vi "Calibration.vi"() -> ()   [LabVIEW 2009]
uses:
  lib/Apps/On Off Button.ctl
  CalibrationRampState.ctl
  Calibration Readings.ctl
  DAQ Read Actions.ctl
  <vilib>/DAQmx/write.llb/DAQmx Write (Analog 1D DBL NChan 1Samp).vi
panel:
  in  "Readings":T1
  in  "Actuator":i32(listbox)
  out "Readings":T2(graph)
  out "Ramp State":T3
  in  "Execute":bool
  in  "Logging":T4
  out "Command Voltage":dbl[](array[numeric])
  in  "Log File Path":path=path "C:/Documents and Settings/mbletzin/Desktop/CalVolts.txt"
  in  "Ramp Voltage":dbl[](array[numeric])
  out "Control Voltage":dbl[](array[numeric])
  in  "rate":dbl=50.0
  in  "samples per channel":i32=30
  out "Servo Error Reading":dbl[](array[numeric])
  in  "Command Voltage Task":refnum<k21>="Command Voltages"
  in  "Readings Task":refnum<k21>="All Readings"
  in  "Write error in (no error)":errorcluster
  out "Read error out":errorcluster
  out "Write error out":errorcluster
  in  "Read error in (no error)":errorcluster
  out "Load Cell \nReading":dbl[](array[numeric])
  out "LVDT Reading":dbl[](array[numeric])
  in  "Command Voltage Input":T5={"Actuator X1"=0.0, "Actuator Z1"=0.0, "Actuator Y1"=0.0, "Actuator X2"=0.0, "Actuator Z3"=0.0, "Actuator Z2"=0.0, "Ramp Time"=30.0, "No. of Steps"=100} {"Actuator Z2" min=-10.0 max=10.0 step=0.1 scale=-10.0..10.0; "Actuator Z3" min=-10.0 max=10.0 step=0.1 scale=-10.0..10.0; "Actuator X2" min=-10.0 max=10.0 step=0.1 scale=-10.0..10.0; "Actuator Y1" min=-10.0 max=10.0 step=0.1 scale=-10.0..10.0; "Actuator Z1" min=-10.0 max=10.0 step=0.1 scale=-10.0..10.0; "Actuator X1" min=-10.0 max=10.0 step=0.1 scale=-10.0..10.0}
  in  "Quit":bool
  # "LBCB CALIBRATION PROGRAM"
  # "Channel Order:\nX1 X2 Y1 Z1 Z2 Z3\n\nLVDT Readings\nLoadcell Readings\nServo Errors"
  # "Channel Order:\nX1 X2 Y1 Z1 Z2 Z3"
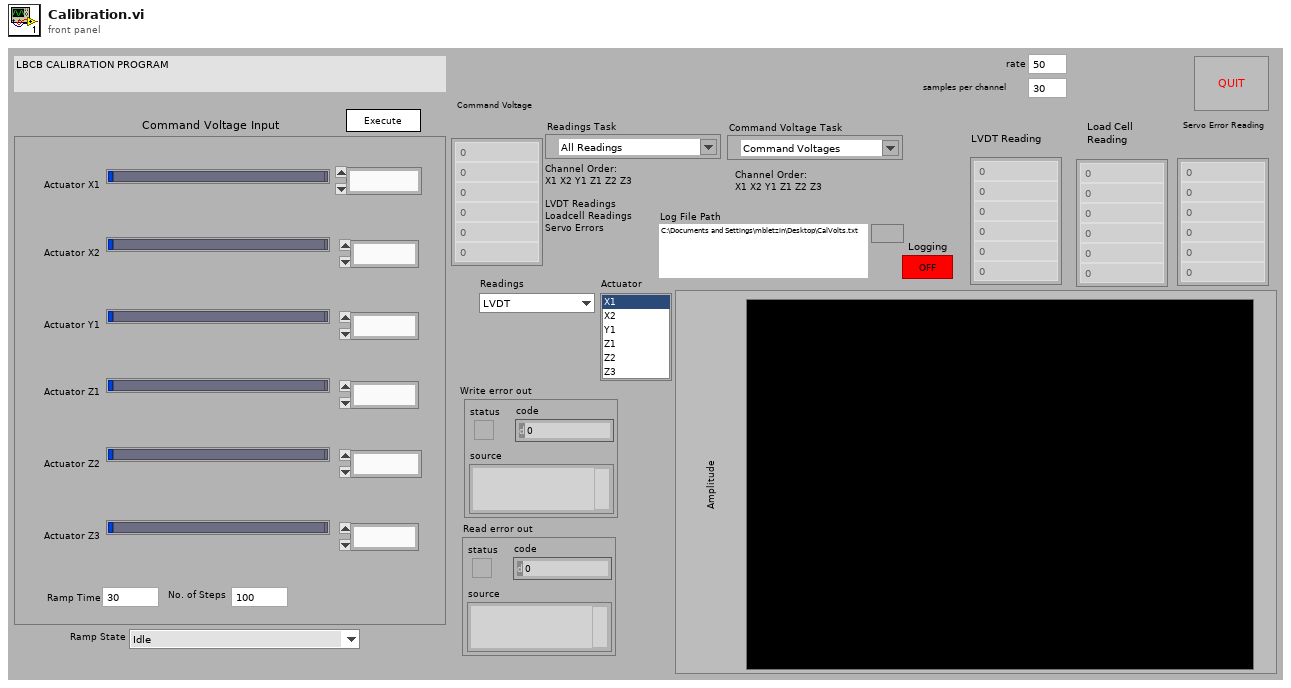
[diagram p1: front panel]
types:
  T1 = typedef "Calibration Readings.ctl" = enum16{"LVDT", "Load Cell", "Servo Errors"}
  T2 = cluster{"Average[0]":dbl, "Average[1]":dbl, "Average[2]":dbl, "Average[3]":dbl, "Average[4]":dbl, "Average[5]":dbl, "Average[6]":dbl, "Average[7]":dbl, "Average[8]":dbl}
  T3 = typedef "CalibrationRampState.ctl" = enum16{"Idle", "Start Ramp", "Ramping"}
  T4 = typedef "On Off Button.ctl" = bool
  T5 = cluster{"Actuator X1":dbl, "Actuator Z1":dbl, "Actuator Y1":dbl, "Actuator X2":dbl, "Actuator Z3":dbl, "Actuator Z2":dbl, "Ramp Time":dbl, "No. of Steps":i32}
  T6 = typedef "DAQ Read Actions.ctl" = enum16{"Start", "Read", "Stop"}
  T7 = cluster{"Average[0]":dbl, "Average[1]":dbl, "Average[2]":dbl, "Average[3]":dbl, "Average[4]":dbl, "Average[5]":dbl, "Average[6]":dbl, "Average[7]":dbl, "Average[8]":dbl}[]
  T8 = enum16{"open", "replace", "create", "open or create", "replace or create", "replace or create with confirmation"}
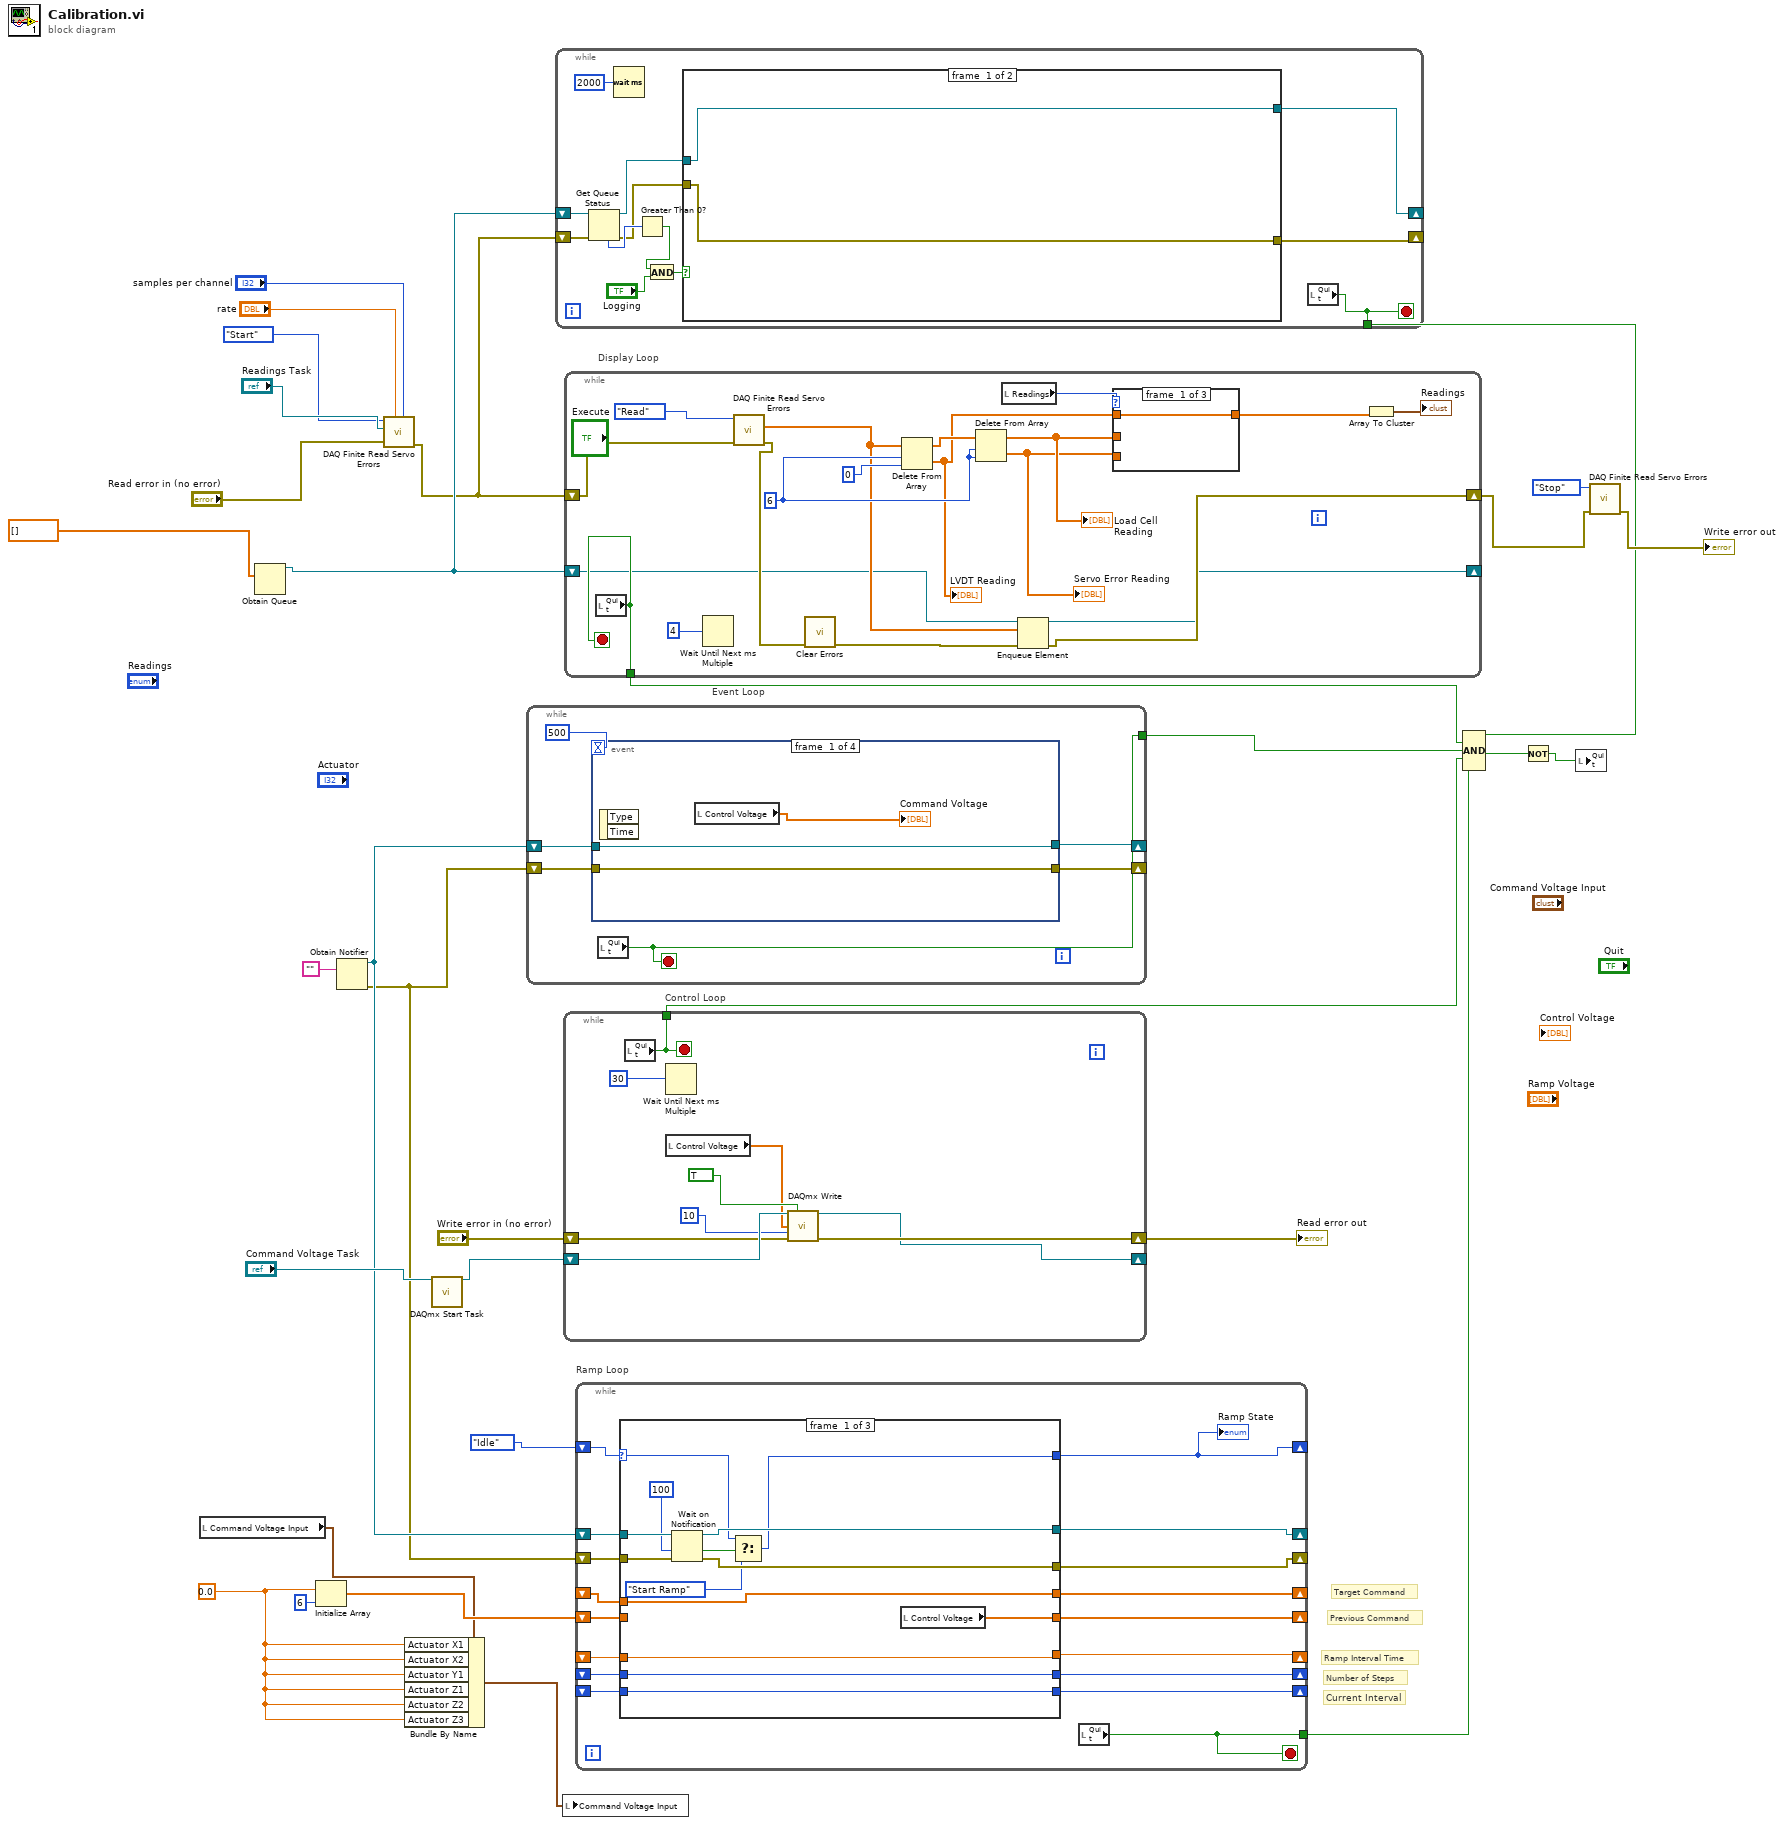
[diagram p0: block diagram]
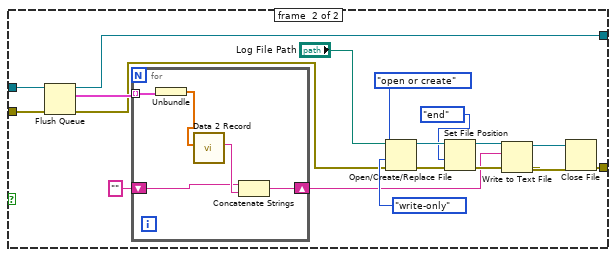
[diagram p2: hidden frame]
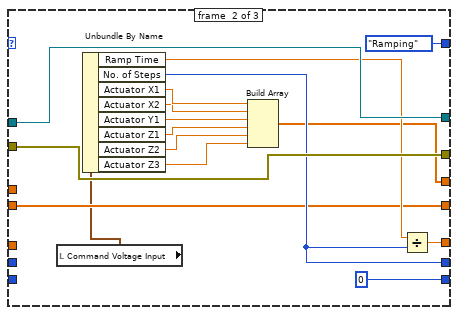
[diagram p3: hidden frame]
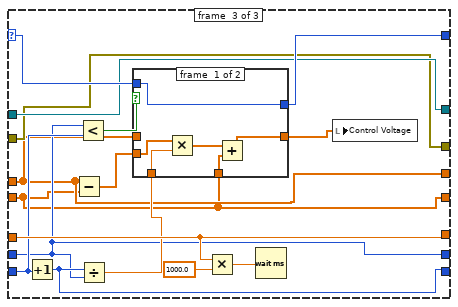
[diagram p4: hidden frame]
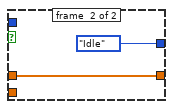
[diagram p5: hidden frame]
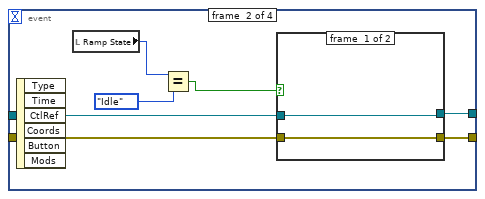
[diagram p6: hidden frame]
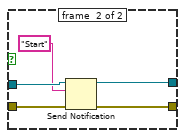
[diagram p7: hidden frame]
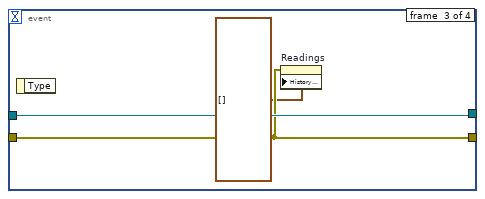
[diagram p8: hidden frame]
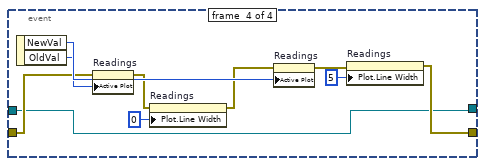
[diagram p9: hidden frame]
diagram:
  w1 = 0.0 ("element")
  # "Previous Command"
  # "Target Command"
  # "Ramp Interval Time"
  # "Number of Steps"
  # "Current Interval"
  n1 = local read "Command Voltage Input"() -> (w2:T5)
  n2 = Obtain Queue(element data type=dbl[] []) -> (queue out=w8:refnum<queue>)  [unwired: 4 in, 2 out]
  n3 = Initialize Array(w1, 6 ("dimension size")) -> (w4:dbl[])
  n4 = Obtain Notifier(notification data type="") -> (notifier out=w12:refnum<notifier>, error out=w11:errorcluster)  [unwired: 3 in, 1 out]
  n5 = call "DAQ Finite Read Servo Errors.vi"("samples per channel"="samples per channel", "rate"="rate", "error in"="Read error in (no error)", "task/channels in"="Readings Task", "Action"=DAQ_Read_Actions."Start") -> ("error out"=w7:errorcluster)  [unwired: 6 out]
  n6 = Bundle By Name(cluster=w2, "Actuator X1"=w1, "Actuator X2"=w1, "Actuator Y1"=w1, "Actuator Z1"=w1, "Actuator Z2"=w1, "Actuator Z3"=w1) -> (w3:T5)
  n7 = call <vilib>:"DAQmx Start Task.vi"("task/channels in"="Command Voltage Task") -> ("task out"=w31:refnum<k21>)  [unwired: 1 in, 13 out]
  n8 = while "Event Loop" {
    tunnel: [w36] -> w27
    shift-right: [w32] -> _
    shift-left: w11 -> [w34]
    shift-right: [w33] -> _
    shift-left: w12 -> [w35]
    stop <- w36 stop-if-true
    n9 = event shown="[2] \"Readings\": Value Change" {
      selector: _ -> [_ _ _ _]
      dyn-events: _ -> [_ _ _ _]
      timeout: 500 -> [_ _ _ _]
      tunnel: w35 -> [w40 w45 w57 w59]
      tunnel: w34 -> [w39 w44 w56 w64]
      tunnel: [w40 w43 w57 w59] -> w33
      tunnel: [w39 w42 w56 w60] -> w32
      event #0 {
        n10 = event-data() -> ()  [unwired: 3 out]
        n11 = local read "Control Voltage"() -> (→"Command Voltage":dbl[])
      }
      event #1 {
        n12 = event-data() -> ()  [unwired: 7 out]
        n13 = local read "Ramp State"() -> (w41:T3)
        n14 = Equal?(x=w41, y=enum16{"Idle", "Start Ramp", "Ramping"}."Idle") -> (x = y?=w46:bool)
        n15 = case shown="True" w46 {
          tunnel: w45 -> [w49 w54]
          tunnel: w44 -> [w48 w52]
          tunnel: [w49 w51] -> w43
          tunnel: [w48 w50] -> w42
          frame #0 {
          }
          frame #1 {
            n16 = Send Notification(notification="Start", notifier=w54, error in (no error)=w52) -> (notifier out=w51:refnum<notifier>, error out=w50:errorcluster)
          }
        }
      }
      event #2 {
        n17 = event-data() -> ()  [unwired: 2 out]
        n18 = property on="Readings" class="WFChart (strict)"(error in=w56, "History Data"=T7 []) -> ()  [unwired: 1 in, 2 out]
      }
      event #3 {
        n19 = event-data() -> ("NewVal"=w67:i32, "OldVal"=w66:i32)  [unwired: 1 out]
        n20 = property on="Readings" class="WFChart (strict)"(error in=w64, "Active Plot"=w66) -> (error out=w65:errorcluster)  [unwired: 1 in, 1 out]
        n21 = property on="Readings" class="WFChart (strict)"(error in=w65, "Plot.Line Width"=u8 0) -> (error out=w62:errorcluster)  [unwired: 1 in, 1 out]
        n22 = property on="Readings" class="WFChart (strict)"(error in=w62, "Active Plot"=w67) -> (error out=w61:errorcluster)  [unwired: 1 in, 1 out]
        n23 = property on="Readings" class="WFChart (strict)"(error in=w61, "Plot.Line Width"=u8 5) -> (error out=w60:errorcluster)  [unwired: 1 in, 1 out]
      }
    }
    n24 = local read "Quit"() -> (w36:bool)
  }
  n25 = while {
    shift-right: [w73] -> _
    shift-left: w8 -> [w79]
    shift-right: [w74] -> _
    shift-left: w7 -> [w78]
    tunnel: [w72] -> w6
    stop <- w72 stop-if-true
    n26 = Get Queue Status(queue=w79, error in (no error)=w78) -> (queue out=w76:refnum<queue>, error out=w75:errorcluster, # elements in queue=w77:i32)  [unwired: 1 in, 5 out]
    n27 = Wait (ms)(milliseconds to wait=u32 2000) -> ()  [unwired: 1 out]
    n28 = Greater Than 0?(x=w77) -> (x > 0?=w69:bool)
    n29 = And(x=w69, y="Logging") -> (x .and. y?=w70:T4)
    n30 = case shown="False" w70 {
      tunnel: w76 -> [w81 w89]
      tunnel: w75 -> [w80 w88]
      tunnel: [w80 w87] -> w74
      tunnel: [w81 w85] -> w73
      frame #0 {
      }
      frame #1 {
        n31 = Flush Queue(queue=w89, error in (no error)=w88) -> (queue out=w85:refnum<queue>, remaining elements=w86:cluster{dbl[]}[], error out=w84:errorcluster)
        n32 = for {
          tunnel: w86 -> [w104] mode=indexing
          shift-right: [w101] -> w83
          shift-left: "" -> [w100]
          n33 = Unbundle(w104) -> (w103:dbl[])
          n34 = call "Data 2 Record.vi"("Data"=w103) -> ("Records"=w102:string)  [unwired: 10 in]
          n35 = Concatenate Strings(w100, w102) -> (w101:string)
        }
        n36 = Open/Create/Replace File(file path (use dialog)="Log File Path", error in=w84, operation (0:open)=T8."open or create", access (0:read/write)=enum16{"read/write", "read-only", "write-only"}."write-only") -> (refnum out=w95:refnum<file>, error out=w94:errorcluster)  [unwired: 3 out]
        n37 = Set File Position(refnum=w95, from (0:start)=enum16{"start", "end", "current"}."end", error in=w94) -> (refnum out=w92:refnum<file>, error out=w93:errorcluster)  [unwired: 1 out]
        n38 = Write to Text File(file (use dialog)=w92, text=w83, error in=w93) -> (refnum out=w97:refnum<file>, error out=w98:errorcluster)  [unwired: 2 out]
        n39 = Close File(refnum=w97, error in=w98) -> (error out=w87:errorcluster)  [unwired: 1 out]
      }
    }
    n40 = local read "Quit"() -> (w72:bool)
  }
  n41 = local write "Command Voltage Input"(w3) -> ()
  n42 = while "Control Loop" {
    shift-right: [w110] -> _
    shift-left: w31 -> [w113]
    shift-right: [w111] -> w29
    shift-left: "Write error in (no error)" -> [w112]
    tunnel: [w106] -> w23
    stop <- w106 stop-if-true
    n43 = local read "Quit"() -> (w106:bool)
    n44 = Wait Until Next ms Multiple(millisecond multiple=30) -> ()  [unwired: 1 out]
    n45 = local read "Control Voltage"() -> (w105:dbl[])
    n46 = call-poly <vilib>:"DAQmx Write.vi"("task/channels in"=w113, "auto start"=TRUE, "data"=w105, "timeout"=10, "error in"=w112) -> ("task out"=w110:refnum<k21>, "error out"=w111:errorcluster)  [unwired: 9 out]
  }
  "Read error out" <- w29
  n47 = while "Display Loop" {
    shift-right: [w123] -> w17
    shift-left: w7 -> [w127]
    tunnel: [w131] -> w25
    shift-right: [w120] -> _
    shift-left: w8 -> [w121]
    stop <- w131 stop-if-true
    w129 = 6
    n48 = local read "Quit"() -> (w131:bool)
    n49 = Wait Until Next ms Multiple(millisecond multiple=4) -> ()  [unwired: 1 out]
    n50 = call "DAQ Finite Read Servo Errors.vi"("error in"=w127, "Action"=DAQ_Read_Actions."Read") -> ("error out"=w126:errorcluster, "Average"=w122:dbl[])  [unwired: 3 in, 5 out]
    n51 = call <vilib>:"Clear Errors.vi"("error in (no error)"=w126) -> ("error out"=w124:errorcluster)  [unwired: 6 out]
    n52 = Delete From Array(array=w122, length=w129, index=0) -> (deleted portion=w118:dbl[], array with subset deleted=w130:dbl[])
    "LVDT Reading" <- w118
    n53 = Delete From Array(array=w130, length=w129, index=w129) -> (deleted portion=w116:dbl[], array with subset deleted=w117:dbl[])
    "Load Cell \nReading" <- w117
    "Servo Error Reading" <- w116
    n54 = local read "Readings"() -> (w119:T1)
    n55 = Enqueue Element(queue=w121, element=w122, error in (no error)=w124) -> (queue out=w120:refnum<queue>, error out=w123:errorcluster)  [unwired: 1 in, 1 out]
    n56 = case shown="\"Servo Errors\"" w119 {
      tunnel: w118 -> [w133 _ _]
      tunnel: w117 -> [_ w134 _]
      tunnel: w116 -> [_ _ w135]
      tunnel: [w133 w134 w135] -> w115
      frame #0 {
      }
      frame #1 {
      }
      frame #2 {
      }
    }
    n57 = Array To Cluster(array=w115) -> (cluster=→"Readings":T2)
  }
  n58 = while "Ramp Loop" {
    shift-right: [w136] -> _
    shift-left: CalibrationRampState."Idle" ("Ramp State") -> [w152]
    shift-right: [w149] -> _
    shift-left: w12 -> [w151]
    shift-right: [w148] -> _
    shift-left: w11 -> [w150]
    shift-right: [w147] -> _
    shift-left: _ -> [w139]
    shift-right: [w145] -> _
    shift-left: _ -> [w140]
    shift-right: [w146] -> _
    shift-left: _ -> [w141]
    shift-right: [w144] -> _
    shift-left: w4 -> [w142]
    shift-right: [w143] -> _
    shift-left: _ -> [w138]
    tunnel: [w137] -> w10
    stop <- w137 stop-if-true
    n59 = case shown="\"Start Ramp\"" w152 {
      selector: w152 -> [w160 _ w188]
      tunnel: w151 -> [w166 w181 w186]
      tunnel: w150 -> [w165 w182 w185]
      tunnel: [w162 w181 w186] -> w149
      tunnel: [w161 w182 w185] -> w148
      tunnel: [w159 CalibrationRampState."Ramping" ("f") w187] -> w136
      tunnel: [w155 w178 w196] -> w147
      tunnel: [w153 0 w195] -> w146
      tunnel: [w154 w176 w189] -> w145
      tunnel: [w157 w168 w183] -> w144
      tunnel: [w156 w169 w184] -> w143
      tunnel: w142 -> [_ w168 w183]
      tunnel: w141 -> [w153 _ w190]
      tunnel: w140 -> [w154 _ w189]
      tunnel: w139 -> [w155 _ w196]
      tunnel: w138 -> [w156 _ w184]
      frame #0 {
        n60 = Wait on Notification(notifier=w166, timeout in ms (-1)=100, error in (no error)=w165) -> (notifier out=w162:refnum<notifier>, timed out?=w163:bool, error out=w161:errorcluster)  [unwired: 1 in, 1 out]
        n61 = Select(t=w160, s=w163, f=CalibrationRampState."Start Ramp") -> (s? t:f=w159:T3)
        n62 = local read "Control Voltage"() -> (w157:dbl[])
      }
      frame #1 {
        n63 = local read "Command Voltage Input"() -> (w167:T5)
        n64 = Unbundle By Name(w167) -> ("Ramp Time"=w179:dbl, "No. of Steps"=w176:i32, "Actuator X1"=w175:dbl, "Actuator X2"=w174:dbl, "Actuator Y1"=w173:dbl, "Actuator Z1"=w172:dbl, "Actuator Z2"=w171:dbl, "Actuator Z3"=w170:dbl)
        n65 = Build Array(w175, w174, w173, w172, w171, w170) -> (w169:dbl[])
        n66 = Divide(x=w179, y=w176) -> (x/y=w178:dbl)
      }
      frame #2 {
        n67 = Increment(x=w190) -> (x+1=w195:i32)
        n68 = Subtract(x=w184, y=w183) -> (x-y=w194:dbl[])
        n69 = Less?(x=w189, y=w190) -> (x < y?=w191:bool)
        n70 = Divide(x=w195, y=w189) -> (x/y=w193:dbl)
        n71 = case shown="False" w191 {
          tunnel: w194 -> [w204 _]
          tunnel: w193 -> [w203 _]
          tunnel: [w200 w205] -> w192
          tunnel: w188 -> [w201 _]
          tunnel: [w201 CalibrationRampState."Idle" ("Ramp State")] -> w187
          tunnel: w184 -> [_ w205]
          tunnel: w183 -> [w199 _]
          frame #0 {
            n72 = Multiply(x=w204, y=w203) -> (x*y=w202:dbl[])
            n73 = Add(x=w202, y=w199) -> (x+y=w200:dbl[])
          }
          frame #1 {
          }
        }
        n74 = Multiply(x=w196, y=1000.0) -> (x*y=w197:dbl)
        n75 = Wait (ms)(milliseconds to wait=w197) -> ()  [unwired: 1 out]
        n76 = local write "Control Voltage"(w192) -> ()
      }
    }
    "Ramp State" <- w136
    n77 = local read "Quit"() -> (w137:bool)
  }
  n78 = Compound Arithmetic op=AND(w6, w25, w27, w23, w10) -> (w26:bool)
  n79 = Not(x=w26) -> (.not. x?=w24:bool)
  n80 = local write "Quit"(w24) -> ()
  n81 = call "DAQ Finite Read Servo Errors.vi"("error in"=w17, "Action"=DAQ_Read_Actions."Stop") -> ("error out"=→"Write error out":errorcluster)  [unwired: 3 in, 6 out]
